vi "dg535 set output.vi"(0 "GPIB address":string="15", 1 "output":u16(ring) items=["T0", "A", "B", "AB", "C", "D", "CD"], 2 "set":bool, 3 "error in":errorcluster, 4 "mode":i32(ring) items=["TTL", "NIM", "ECL", "VAR"], 5 "offset":dbl min=-3.0 max=4.0 format="%.2f", 6 "amplitude":dbl=1.0 min=-3.0 max=4.0 format="%.2f", 7 "inversion":bool, 8 "load":bool) -> (9 "error out":errorcluster)   [LabVIEW 2013]
doc: "This subVI sets the mode , load , output polarity , amplitude and offset of an output BNC .\nOUTPUT selects the BNC whose parameters will be changed .\nMODE specifies the output mode to be one of TTL, NIM , ECL or VAR .\nLOAD configures the output to drive either a 50 Ohm load or a High Z load .\nINVERSION sets the polarity of logic pulses at the BNC outputs. \nAMPLITUDE and OFFSET set the size of the step and the offset of the output BNCs when in the VARiable mode ."
panel:
  # "50 Ohm\nHigh Z"
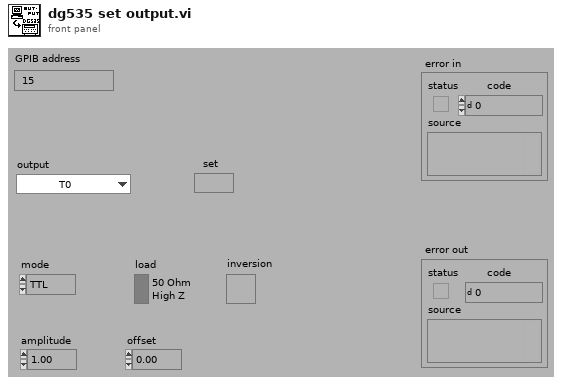
[diagram p1: front panel]
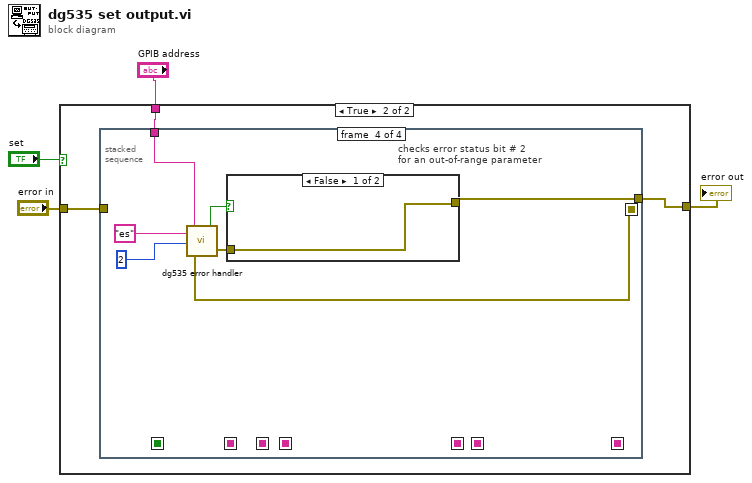
[diagram p0: block diagram]
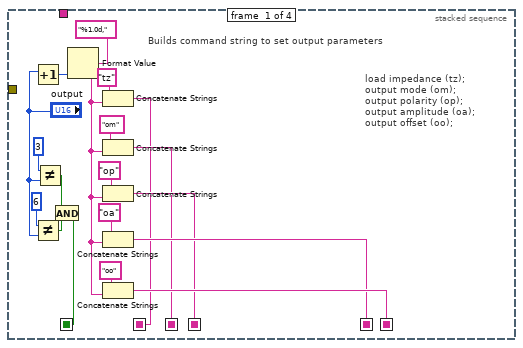
[diagram p3: hidden frame]
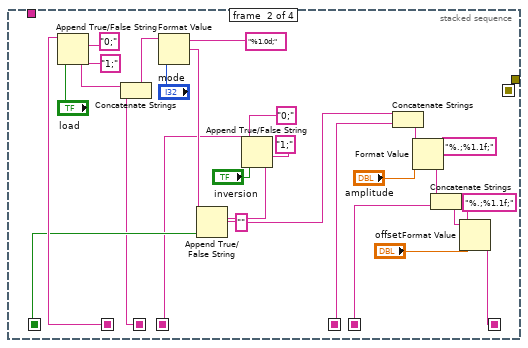
[diagram p4: hidden frame]
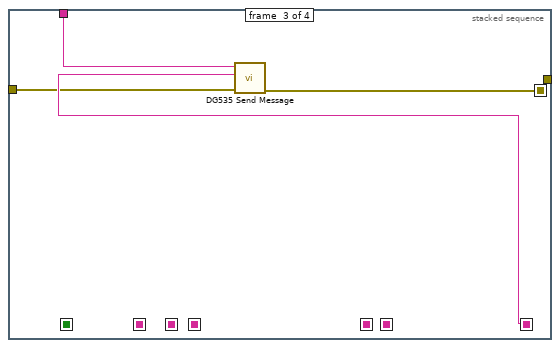
[diagram p5: hidden frame]
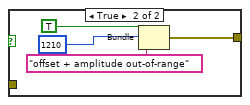
[diagram p6: hidden frame]
diagram:
  n1 = case shown="True" "set" {
    tunnel: "GPIB address" -> [_ w8]
    tunnel: "error in" -> [w5 w7]
    tunnel: [w5 w6] -> w1
    frame False {
      # "Exits the subVI if SET is off"
    }
    frame True {
      n2 = stacked-sequence {
        seq-local: [w20 _ _ _] -> [_ w33 _ _]
        seq-local: [w19 _ _ _] -> [_ w37 _ _]
        seq-local: [w18 _ _ _] -> [_ w34 _ _]
        seq-local: [w17 _ _ _] -> [_ w55 _ _]
        seq-local: [w21 _ _ _] -> [_ w43 _ _]
        seq-local: [w11 _ _ _] -> [_ w38 _ _]
        seq-local: [_ w31 _ _] -> [_ _ w58 _]
        seq-local: [_ _ w57 _] -> [_ _ _ w61]
        tunnel: w8 -> [_ _ w59 w62]
        tunnel: w7 -> [_ _ w56 _]
        tunnel: [_ _ _ w60] -> w6
        frame #0 {
          # "load impedance (tz);\noutput mode (om);\noutput polarity (op);\noutput amplitude (oa);\noutput offset (oo);"
          # "Builds command string to set output parameters"
          n3 = Increment(x="output") -> (x+1=w16:u16)
          n4 = Not Equal?(x=6, y="output") -> (x != y?=w12:bool)
          n5 = Not Equal?(x=3, y="output") -> (x != y?=w13:bool)
          n6 = And(x=w13, y=w12) -> (x .and. y?=w11:bool)
          n7 = Format Value(format string="%1.0d,", value (0)=w16) -> (output string=w9:string)  [unwired: 1 in]
          n8 = Concatenate Strings("tz", w9) -> (w17:string)
          n9 = Concatenate Strings("om", w9) -> (w18:string)
          n10 = Concatenate Strings("op", w9) -> (w19:string)
          n11 = Concatenate Strings("oa", w9) -> (w20:string)
          n12 = Concatenate Strings("oo", w9) -> (w21:string)
        }
        frame #1 {
          n13 = Append True/False String(1:"load", 2:"1;", 3:"0;", 4:w55) -> (0:w50:string)
          n14 = Concatenate Strings(w50, w34) -> (w49:string)
          n15 = Format Value(string ("")=w49, format string="%1.0d;", value (0)="mode") -> (output string=w39:string)
          n16 = Append True/False String(1:"inversion", 2:"1;", 3:"0;", 4:w37) -> (0:w36:string)
          n17 = Append True/False String(1:w38, 2:"", 3:w36, 4:w39) -> (0:w32:string)
          n18 = Concatenate Strings(w32, w33) -> (w45:string)
          n19 = Format Value(string ("")=w45, format string="%.;%1.1f;", value (0)="amplitude") -> (output string=w42:string)
          n20 = Concatenate Strings(w42, w43) -> (w41:string)
          n21 = Format Value(string ("")=w41, format string="%.;%1.1f;", value (0)="offset") -> (output string=w31:string)
        }
        frame #2 {
          n22 = call "DG535 Send Message.vi"("address string"=w59, "write buffer"=w58, "error in"=w56) -> ("error out"=w57:errorcluster)  [unwired: 4 in, 2 out]
        }
        frame #3 {
          # "checks error status bit # 2\nfor an out-of-range parameter"
          n23 = call "dg535 error handler.vi"("error in"=w61, "check bit #"=2, "command string"="es", "GPIB address"=w62) -> ("error out"=w63:errorcluster, "error found"=w64:bool)
          n24 = case shown="False" w64 {
            tunnel: [w67 w68] -> w60
            tunnel: w63 -> [w67 _]
            frame False {
            }
            frame True {
              n25 = Bundle(TRUE, 1210, "offset + amplitude out-of-range") -> (w68:errorcluster)  [unwired: 1 in]
            }
          }
        }
      }
    }
  }
  "error out" <- w1
